vi "Setup.vi"(6 "Open Block Diagram?":bool=TRUE, 8 "Error In":errorcluster, 11 "VI In":refnum<vi>) -> (0 "Error Out":errorcluster, 3 "VI Out":refnum<vi>)   [LabVIEW 2018, in "Tests.lvlib"]
doc: "Sets up a test."
uses:
  Tests.lvlib
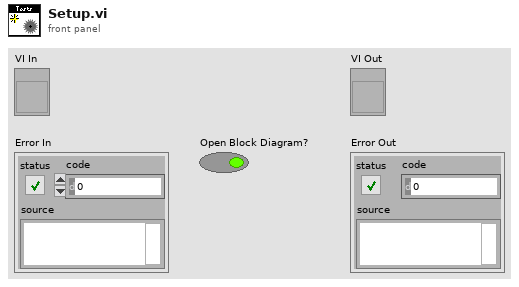
[diagram p1: front panel]
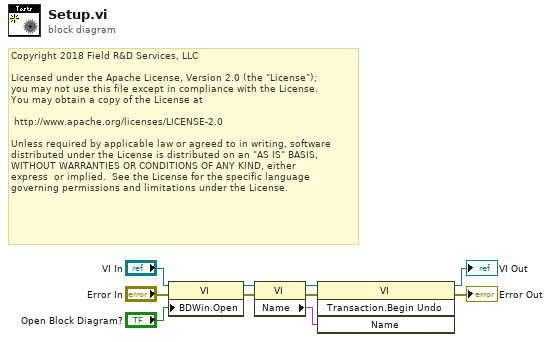
[diagram p0: block diagram]
diagram:
  # "Copyright 2018 Field R&D Services, LLC\n\nLicensed under the Apache License, Version 2.0 (the \"License\");\nyou may not use this file except in compliance with the License.\nYou may obtain a copy of the License at\n\n\thttp://www.apache.org/licenses/LICENSE-2.0\n\nUnless required by applicable law or agreed to in writing, software\ndistributed under the License is distributed on an \"AS IS\" BASIS,\nWITHOUT WARRANTIES OR CONDITIONS OF ANY KIND, either \nexpress  or implied.  See the License for the specific language \ngoverning permissions and limitations under the License."
  n1 = property class="VI"(reference="VI In", error in="Error In", "BDWin.Open"="Open Block Diagram?") -> (reference out=w7:refnum<vi>, error out=w3:errorcluster)
  n2 = property class="VI"(reference=w7, error in=w3) -> (reference out=w4:refnum<vi>, error out=w2:errorcluster, "Name"=w1:string)
  n3 = invoke class="VI" method="Transaction.Begin Undo"(reference=w4, error in=w2, "Name"=w1) -> (reference out=→"VI Out":refnum<vi>, error out=→"Error Out":errorcluster)  [unwired: 1 in, 2 out]
